vi "Swerve Conv (SubVI).vi"() -> (0 "steeringModuleCPR":dbl, 1 "driveCountsPerMeter":dbl, 2 "driveCountsPerInch":dbl, 3 "steeringModuleCPD":dbl)   [LabVIEW 2020]
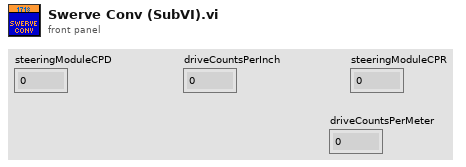
[diagram p1: front panel]
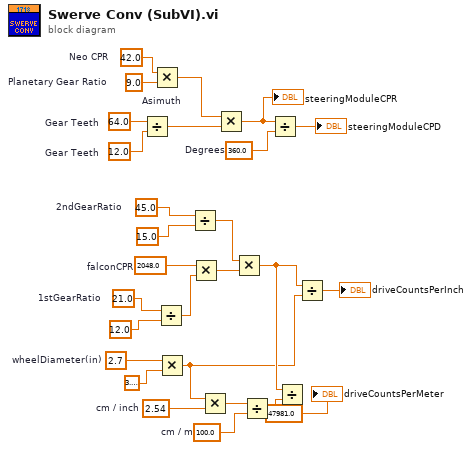
[diagram p0: block diagram]
diagram:
  w6 = 100.0  # cm / m
  w8 = 2.54  # cm / inch
  w11 = 2.7  # wheelDiameter(in)
  w2 = 45.0  # 2ndGearRatio
  w17 = 21.0  # 1stGearRatio
  w18 = 2048.0  # falconCPR
  w25 = 360.0  # Degrees
  w24 = 12.0  # Gear Teeth
  w23 = 64.0  # Gear Teeth
  w20 = 9.0  # Planetary Gear Ratio
  w19 = 42.0  # Neo CPR
  n1 = Divide "Asimuth"(x=w23, y=w24) -> (x/y=w22:dbl)
  n2 = Multiply(x=w19, y=w20) -> (x*y=w21:dbl)
  n3 = Divide(x=w17, y=12.0) -> (x/y=w15:dbl)
  n4 = Multiply(x=w11, y=3.141592653589793) -> (x*y=w3:dbl)
  n5 = Divide(x=w2, y=15.0) -> (x/y=w12:dbl)
  n6 = Multiply(x=w18, y=w15) -> (x*y=w13:dbl)
  n7 = Multiply(x=w3, y=w8) -> (x*y=w7:dbl)
  n8 = Multiply(x=w21, y=w22) -> (x*y=w27:dbl)
  "steeringModuleCPR" <- w27
  n9 = Multiply(x=w12, y=w13) -> (x*y=w4:dbl)
  n10 = Divide(x=w7, y=w6) -> (x/y=w5:dbl)
  n11 = Divide(x=w27, y=w25) -> (x/y=→"steeringModuleCPD":dbl)
  n12 = Divide(x=w4, y=w5) -> ()  [unwired: 1 out]
  n13 = Divide(x=w4, y=w3) -> (x/y=→"driveCountsPerInch":dbl)
  "driveCountsPerMeter" <- 47981.0 ("driveCountsPerMeter")
